vi "Configure Resistor Voltage Coefficient Test.vi"(6 "Resistor Bias Voltage2 (2)":dbl=2.0, 7 "Resistor Bias Voltage1 (1)":dbl=1.0, 8 "error in (no error)":errorcluster, 9 "Resistor Measure Delay2 (1)":dbl=1.0, 10 "Resistor Measure Delay1 (1)":dbl=1.0, 11 "VISA resource name":refnum<visa-resource-name>) -> (0 "error out":errorcluster, 3 "VISA resource name out":refnum<visa-resource-name>)   [LabVIEW 2020, in "Keithley 6517.lvlib"]
doc: "Sets the resistor voltage coefficient test.\n\nNote:\nCall <b> Configure Test Sequence Common Characteristics </b> first to arm and configures the test sequence.\n\nThis VI is <B>NOT</B> compatible with model <B>6514</B>."
uses:
  <instrlib>/Keithley 6517/Keithley 6517.lvlib
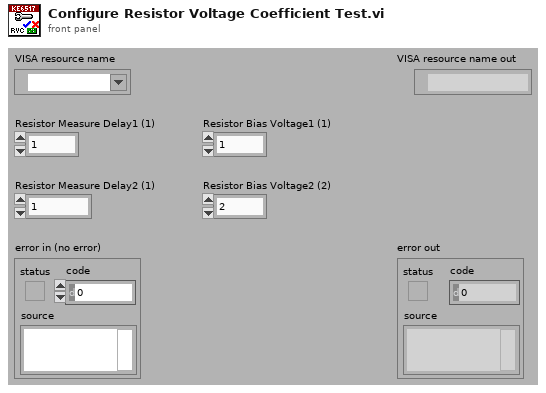
[diagram p1: front panel]
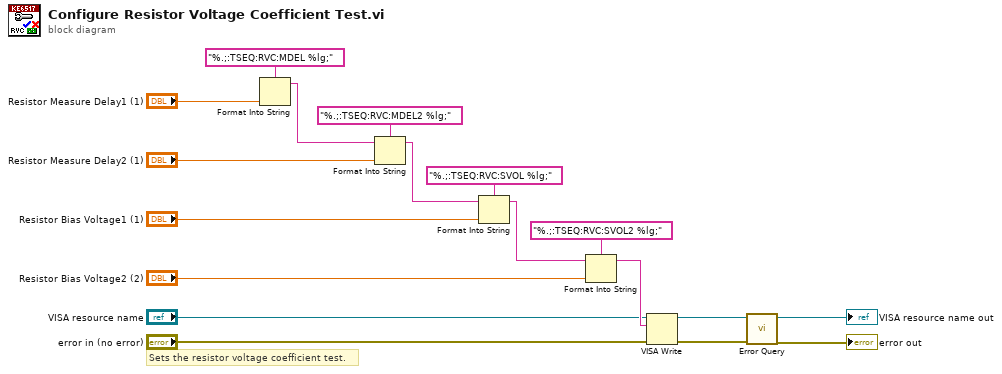
[diagram p0: block diagram]
diagram:
  # "Sets the resistor voltage coefficient test."
  n1 = Format Into String(format string="%.;:TSEQ:RVC:MDEL %lg;", "Resistor Measure Delay1 (1)") -> (resulting string=w16:string)  [unwired: 2 in, 1 out]
  n2 = Format Into String(format string="%.;:TSEQ:RVC:MDEL2 %lg;", initial string=w16, "Resistor Measure Delay2 (1)") -> (resulting string=w13:string)  [unwired: 1 in, 1 out]
  n3 = Format Into String(format string="%.;:TSEQ:RVC:SVOL %lg;", initial string=w13, "Resistor Bias Voltage1 (1)") -> (resulting string=w10:string)  [unwired: 1 in, 1 out]
  n4 = Format Into String(format string="%.;:TSEQ:RVC:SVOL2 %lg;", initial string=w10, "Resistor Bias Voltage2 (2)") -> (resulting string=w7:string)  [unwired: 1 in, 1 out]
  n5 = VISA Write(VISA resource name="VISA resource name", write buffer=w7, error in (no error)="error in (no error)") -> (VISA resource name out=w4:refnum<visa-resource-name>, error out=w3:errorcluster)  [unwired: 1 out]
  n6 = call <instrlib>:"Error Query.vi"("error in (no error)"=w3, "VISA resource name"=w4) -> ("error out"=→"error out":errorcluster, "VISA resource name out"=→"VISA resource name out":refnum<visa-resource-name>)  [unwired: 6 in, 2 out]
